vi "DSA Configure AI and AO.vi"(0 "Input  Physical Channel":tag[](array[tag]), 1 "Output Physical Channel":tag[](array[tag]), 2 "Settings Cluster":T1={"Supply Voltage [Vdc]"=0.0, "Max Supply Current [Idc]"=0.0, "Settling Delay"=0.0, "Temp Criteria"=0.0, "Voltage Steps [Vrms]"=[], "User Notes"="", "Config Wave File Path"=path "", "Config Voltage [Vrms]"=0.0, "Channel Configuration List"={"Channel Configuration Cluster"={"Input"=enum."---", "Enable"=FALSE, "User Notes"="", "Voltage Range"=0.0, "Current Range"=2.5}, "Channel Configuration Cluster 2"={"Input"=enum."---", "Enable"=FALSE, "User Notes"="", "Voltage Range"=0.0, "Current Range"=2.5}, "Channel Configuration Cluster 3"={"Input"=enum."---", "Enable"=FALSE, "User Notes"="", "Voltage Range"=0.0, "Current Range"=2.5}, "Channel Configuration Cluster 4"={"Input"=enum."---", "Enable"=FALSE, "User Notes"="", "Voltage Range"=0.0, "Current Range"=2.5}, "Channel Configuration Cluster 5"={"Input"=enum."---", "Enable"=FALSE, "User Notes"="", "Voltage Range"=0.0, "Current Range"=2.5}, "Channel Configuration Cluster 6"={"Input"=enum."---", "Enable"=FALSE, "User Notes"="", "Voltage Range"=0.0, "Current Range"=2.5}, "Channel Configuration Cluster 7"={"Input"=enum."---", "Enable"=FALSE, "User Notes"="", "Voltage Range"=0.0, "Current Range"=2.5}, "Channel Configuration Cluster 8"={"Input"=enum."---", "Enable"=FALSE, "User Notes"="", "Voltage Range"=0.0, "Current Range"=2.5}, "Channel Configuration Cluster 9"={"Input"=enum."---", "Enable"=FALSE, "User Notes"="", "Voltage Range"=0.0, "Current Range"=2.5}, "Channel Configuration Cluster 10"={"Input"=enum."---", "Enable"=FALSE, "User Notes"="", "Voltage Range"=0.0, "Current Range"=2.5}, "Channel Configuration Cluster 11"={"Input"=enum."---", "Enable"=FALSE, "User Notes"="", "Voltage Range"=0.0, "Current Range"=2.5}, "Channel Configuration Cluster 12"={"Input"=enum."---", "Enable"=FALSE, "User Notes"="", "Voltage Range"=0.0, "Current Range"=2.5}, "Channel Configuration Cluster 13"={"Input"=enum."---", "Enable"=FALSE, "User Notes"="", "Voltage Range"=0.0, "Current Range"=2.5}, "Channel Configuration Cluster 14"={"Input"=enum."---", "Enable"=FALSE, "User Notes"="", "Voltage Range"=0.0, "Current Range"=2.5}, "Channel Configuration Cluster 15"={"Input"=enum."---", "Enable"=FALSE, "User Notes"="", "Voltage Range"=0.0, "Current Range"=2.5}, "Channel Configuration Cluster 16"={"Input"=enum."---", "Enable"=FALSE, "User Notes"="", "Voltage Range"=0.0, "Current Range"=2.5}, "Channel Configuration Cluster 17"={"Input"=enum."---", "Enable"=FALSE, "User Notes"="", "Voltage Range"=0.0, "Current Range"=2.5}}, "User Gains"={"Gain 1"=0.0, "Gain 2"=0.0, "Gain 3"=0.0, "Gain 4"=0.0, "Gain 5"=0.0, "Gain 6"=0.0}, "Gains"={"Gain 1"=0.0, "Gain 2"=0.0, "Gain 3"=0.0, "Gain 4"=0.0, "Gain 5"=0.0, "Gain 6"=0.0}, "Gain Array"={"Gain 1"=0.0, "Gain 2"=0.0, "Gain 3"=0.0, "Gain 4"=0.0, "Gain 5"=0.0, "Gain 6"=0.0, "Gain 7"=0.0, "Gain 8"=0.0, "Gain 9"=0.0, "Gain 10"=0.0, "Gain 11"=0.0, "Gain 12"=0.0, "Gain 13"=0.0, "Gain 14"=0.0, "Gain 15"=0.0, "Gain 16"=0.0, "Gain 17"=0.0}, "Wave File Path 1"=path "", "Wave File Path 2"=path "", "Wave File Path 3"=path "", "Wave File Path 4"=path "", "Range"=FALSE, "CF"=FALSE} {"Gain Array"."Gain 17" format="%.2f"; "Gain Array"."Gain 16" format="%.2f"; "Gain Array"."Gain 15" format="%.2f"; "Gain Array"."Gain 14" format="%.2f"; "Gain Array"."Gain 13" format="%.2f"; "Gain Array"."Gain 12" format="%.2f"; "Gain Array"."Gain 11" format="%.2f"; "Gain Array"."Gain 10" format="%.2f"; "Gain Array"."Gain 9" format="%.2f"; "Gain Array"."Gain 8" format="%.2f"; "Gain Array"."Gain 7" format="%.2f"; "Gain Array"."Gain 6" format="%.2f"; "Gain Array"."Gain 5" format="%.2f"; "Gain Array"."Gain 4" format="%.2f"; "Gain Array"."Gain 3" format="%.2f"; "Gain Array"."Gain 2" format="%.2f"; "Gain Array"."Gain 1" format="%.2f"; "Gains"."Gain 6" format="%.2f"; "Gains"."Gain 5" format="%.2f"; "Gains"."Gain 4" format="%.2f"; "Gains"."Gain 3" format="%.2f"; "Gains"."Gain 2" format="%.2f"; "Gains"."Gain 1" format="%.2f"; "User Gains"."Gain 6" format="%.2f"; "User Gains"."Gain 5" format="%.2f"; "User Gains"."Gain 4" format="%.2f"; "User Gains"."Gain 3" format="%.2f"; "User Gains"."Gain 2" format="%.2f"; "User Gains"."Gain 1" format="%.2f"; "Channel Configuration List"."Channel Configuration Cluster 17"."Current Range" items=["1 <500m>"=0.5, "2 <1>"=1.0, "5 <2.5>"=2.5, "10 <5>"=5.0, "20 <10>"=10.0, "50 <25>"=25.0]; "Channel Configuration List"."Channel Configuration Cluster 17"."Voltage Range" items=["1.5 <0.75>"=0.75, "3 <1.5>"=1.5, "6 <3>"=3.0, "10 <5>"=5.0, "15 <7.5>"=7.5, "30 <15>"=15.0, "60 <30>"=30.0, "100 <50>"=50.0, "150 <75>"=75.0, "300 <150>"=150.0, "600 <300>"=300.0, "1000 <500>"=500.0]; "Channel Configuration List"."Channel Configuration Cluster 16"."Current Range" items=["1 <500m>"=0.5, "2 <1>"=1.0, "5 <2.5>"=2.5, "10 <5>"=5.0, "20 <10>"=10.0, "50 <25>"=25.0]; "Channel Configuration List"."Channel Configuration Cluster 16"."Voltage Range" items=["1.5 <0.75>"=0.75, "3 <1.5>"=1.5, "6 <3>"=3.0, "10 <5>"=5.0, "15 <7.5>"=7.5, "30 <15>"=15.0, "60 <30>"=30.0, "100 <50>"=50.0, "150 <75>"=75.0, "300 <150>"=150.0, "600 <300>"=300.0, "1000 <500>"=500.0]; "Channel Configuration List"."Channel Configuration Cluster 15"."Current Range" items=["1 <500m>"=0.5, "2 <1>"=1.0, "5 <2.5>"=2.5, "10 <5>"=5.0, "20 <10>"=10.0, "50 <25>"=25.0]; "Channel Configuration List"."Channel Configuration Cluster 15"."Voltage Range" items=["1.5 <0.75>"=0.75, "3 <1.5>"=1.5, "6 <3>"=3.0, "10 <5>"=5.0, "15 <7.5>"=7.5, "30 <15>"=15.0, "60 <30>"=30.0, "100 <50>"=50.0, "150 <75>"=75.0, "300 <150>"=150.0, "600 <300>"=300.0, "1000 <500>"=500.0]; "Channel Configuration List"."Channel Configuration Cluster 14"."Current Range" items=["1 <500m>"=0.5, "2 <1>"=1.0, "5 <2.5>"=2.5, "10 <5>"=5.0, "20 <10>"=10.0, "50 <25>"=25.0]; "Channel Configuration List"."Channel Configuration Cluster 14"."Voltage Range" items=["1.5 <0.75>"=0.75, "3 <1.5>"=1.5, "6 <3>"=3.0, "10 <5>"=5.0, "15 <7.5>"=7.5, "30 <15>"=15.0, "60 <30>"=30.0, "100 <50>"=50.0, "150 <75>"=75.0, "300 <150>"=150.0, "600 <300>"=300.0, "1000 <500>"=500.0]; "Channel Configuration List"."Channel Configuration Cluster 13"."Current Range" items=["1 <500m>"=0.5, "2 <1>"=1.0, "5 <2.5>"=2.5, "10 <5>"=5.0, "20 <10>"=10.0, "50 <25>"=25.0]; "Channel Configuration List"."Channel Configuration Cluster 13"."Voltage Range" items=["1.5 <0.75>"=0.75, "3 <1.5>"=1.5, "6 <3>"=3.0, "10 <5>"=5.0, "15 <7.5>"=7.5, "30 <15>"=15.0, "60 <30>"=30.0, "100 <50>"=50.0, "150 <75>"=75.0, "300 <150>"=150.0, "600 <300>"=300.0, "1000 <500>"=500.0]; "Channel Configuration List"."Channel Configuration Cluster 12"."Current Range" items=["1 <500m>"=0.5, "2 <1>"=1.0, "5 <2.5>"=2.5, "10 <5>"=5.0, "20 <10>"=10.0, "50 <25>"=25.0]; "Channel Configuration List"."Channel Configuration Cluster 12"."Voltage Range" items=["1.5 <0.75>"=0.75, "3 <1.5>"=1.5, "6 <3>"=3.0, "10 <5>"=5.0, "15 <7.5>"=7.5, "30 <15>"=15.0, "60 <30>"=30.0, "100 <50>"=50.0, "150 <75>"=75.0, "300 <150>"=150.0, "600 <300>"=300.0, "1000 <500>"=500.0]; "Channel Configuration List"."Channel Configuration Cluster 11"."Current Range" items=["1 <500m>"=0.5, "2 <1>"=1.0, "5 <2.5>"=2.5, "10 <5>"=5.0, "20 <10>"=10.0, "50 <25>"=25.0]; "Channel Configuration List"."Channel Configuration Cluster 11"."Voltage Range" items=["1.5 <0.75>"=0.75, "3 <1.5>"=1.5, "6 <3>"=3.0, "10 <5>"=5.0, "15 <7.5>"=7.5, "30 <15>"=15.0, "60 <30>"=30.0, "100 <50>"=50.0, "150 <75>"=75.0, "300 <150>"=150.0, "600 <300>"=300.0, "1000 <500>"=500.0]; "Channel Configuration List"."Channel Configuration Cluster 10"."Current Range" items=["1 <500m>"=0.5, "2 <1>"=1.0, "5 <2.5>"=2.5, "10 <5>"=5.0, "20 <10>"=10.0, "50 <25>"=25.0]; "Channel Configuration List"."Channel Configuration Cluster 10"."Voltage Range" items=["1.5 <0.75>"=0.75, "3 <1.5>"=1.5, "6 <3>"=3.0, "10 <5>"=5.0, "15 <7.5>"=7.5, "30 <15>"=15.0, "60 <30>"=30.0, "100 <50>"=50.0, "150 <75>"=75.0, "300 <150>"=150.0, "600 <300>"=300.0, "1000 <500>"=500.0]; "Channel Configuration List"."Channel Configuration Cluster 9"."Voltage Range" items=["1.5 <0.75>"=0.75, "3 <1.5>"=1.5, "6 <3>"=3.0, "10 <5>"=5.0, "15 <7.5>"=7.5, "30 <15>"=15.0, "60 <30>"=30.0, "100 <50>"=50.0, "150 <75>"=75.0, "300 <150>"=150.0, "600 <300>"=300.0, "1000 <500>"=500.0]; "Channel Configuration List"."Channel Configuration Cluster 9"."Current Range" items=["10m <5m>"=0.005, "20m <10m>"=0.01, "50m <25m>"=0.025, "100m <50m>"=0.05, "200m <100m>"=0.1, "500m <250m>"=0.25, "1 <500m>"=0.5, "2 <1>"=1.0, "5 <2.5>"=2.5]; "Channel Configuration List"."Channel Configuration Cluster 8"."Voltage Range" items=["1.5 <0.75>"=0.75, "3 <1.5>"=1.5, "6 <3>"=3.0, "10 <5>"=5.0, "15 <7.5>"=7.5, "30 <15>"=15.0, "60 <30>"=30.0, "100 <50>"=50.0, "150 <75>"=75.0, "300 <150>"=150.0, "600 <300>"=300.0, "1000 <500>"=500.0]; "Channel Configuration List"."Channel Configuration Cluster 8"."Current Range" items=["10m <5m>"=0.005, "20m <10m>"=0.01, "50m <25m>"=0.025, "100m <50m>"=0.05, "200m <100m>"=0.1, "500m <250m>"=0.25, "1 <500m>"=0.5, "2 <1>"=1.0, "5 <2.5>"=2.5]; "Channel Configuration List"."Channel Configuration Cluster 7"."Voltage Range" items=["1.5 <0.75>"=0.75, "3 <1.5>"=1.5, "6 <3>"=3.0, "10 <5>"=5.0, "15 <7.5>"=7.5, "30 <15>"=15.0, "60 <30>"=30.0, "100 <50>"=50.0, "150 <75>"=75.0, "300 <150>"=150.0, "600 <300>"=300.0, "1000 <500>"=500.0]; "Channel Configuration List"."Channel Configuration Cluster 7"."Current Range" items=["10m <5m>"=0.005, "20m <10m>"=0.01, "50m <25m>"=0.025, "100m <50m>"=0.05, "200m <100m>"=0.1, "500m <250m>"=0.25, "1 <500m>"=0.5, "2 <1>"=1.0, "5 <2.5>"=2.5]; "Channel Configuration List"."Channel Configuration Cluster 6"."Voltage Range" items=["1.5 <0.75>"=0.75, "3 <1.5>"=1.5, "6 <3>"=3.0, "10 <5>"=5.0, "15 <7.5>"=7.5, "30 <15>"=15.0, "60 <30>"=30.0, "100 <50>"=50.0, "150 <75>"=75.0, "300 <150>"=150.0, "600 <300>"=300.0, "1000 <500>"=500.0]; "Channel Configuration List"."Channel Configuration Cluster 6"."Current Range" items=["10m <5m>"=0.005, "20m <10m>"=0.01, "50m <25m>"=0.025, "100m <50m>"=0.05, "200m <100m>"=0.1, "500m <250m>"=0.25, "1 <500m>"=0.5, "2 <1>"=1.0, "5 <2.5>"=2.5]; "Channel Configuration List"."Channel Configuration Cluster 5"."Voltage Range" items=["1.5 <0.75>"=0.75, "3 <1.5>"=1.5, "6 <3>"=3.0, "10 <5>"=5.0, "15 <7.5>"=7.5, "30 <15>"=15.0, "60 <30>"=30.0, "100 <50>"=50.0, "150 <75>"=75.0, "300 <150>"=150.0, "600 <300>"=300.0, "1000 <500>"=500.0]; "Channel Configuration List"."Channel Configuration Cluster 5"."Current Range" items=["10m <5m>"=0.005, "20m <10m>"=0.01, "50m <25m>"=0.025, "100m <50m>"=0.05, "200m <100m>"=0.1, "500m <250m>"=0.25, "1 <500m>"=0.5, "2 <1>"=1.0, "5 <2.5>"=2.5]; "Channel Configuration List"."Channel Configuration Cluster 4"."Voltage Range" items=["1.5 <0.75>"=0.75, "3 <1.5>"=1.5, "6 <3>"=3.0, "10 <5>"=5.0, "15 <7.5>"=7.5, "30 <15>"=15.0, "60 <30>"=30.0, "100 <50>"=50.0, "150 <75>"=75.0, "300 <150>"=150.0, "600 <300>"=300.0, "1000 <500>"=500.0]; "Channel Configuration List"."Channel Configuration Cluster 4"."Current Range" items=["10m <5m>"=0.005, "20m <10m>"=0.01, "50m <25m>"=0.025, "100m <50m>"=0.05, "200m <100m>"=0.1, "500m <250m>"=0.25, "1 <500m>"=0.5, "2 <1>"=1.0, "5 <2.5>"=2.5]; "Channel Configuration List"."Channel Configuration Cluster 3"."Voltage Range" items=["1.5 <0.75>"=0.75, "3 <1.5>"=1.5, "6 <3>"=3.0, "10 <5>"=5.0, "15 <7.5>"=7.5, "30 <15>"=15.0, "60 <30>"=30.0, "100 <50>"=50.0, "150 <75>"=75.0, "300 <150>"=150.0, "600 <300>"=300.0, "1000 <500>"=500.0]; "Channel Configuration List"."Channel Configuration Cluster 3"."Current Range" items=["10m <5m>"=0.005, "20m <10m>"=0.01, "50m <25m>"=0.025, "100m <50m>"=0.05, "200m <100m>"=0.1, "500m <250m>"=0.25, "1 <500m>"=0.5, "2 <1>"=1.0, "5 <2.5>"=2.5]; "Channel Configuration List"."Channel Configuration Cluster 2"."Voltage Range" items=["1.5 <0.75>"=0.75, "3 <1.5>"=1.5, "6 <3>"=3.0, "10 <5>"=5.0, "15 <7.5>"=7.5, "30 <15>"=15.0, "60 <30>"=30.0, "100 <50>"=50.0, "150 <75>"=75.0, "300 <150>"=150.0, "600 <300>"=300.0, "1000 <500>"=500.0]; "Channel Configuration List"."Channel Configuration Cluster 2"."Current Range" items=["10m <5m>"=0.005, "20m <10m>"=0.01, "50m <25m>"=0.025, "100m <50m>"=0.05, "200m <100m>"=0.1, "500m <250m>"=0.25, "1 <500m>"=0.5, "2 <1>"=1.0, "5 <2.5>"=2.5]; "Channel Configuration List"."Channel Configuration Cluster"."Voltage Range" items=["1.5 <0.75>"=0.75, "3 <1.5>"=1.5, "6 <3>"=3.0, "10 <5>"=5.0, "15 <7.5>"=7.5, "30 <15>"=15.0, "60 <30>"=30.0, "100 <50>"=50.0, "150 <75>"=75.0, "300 <150>"=150.0, "600 <300>"=300.0, "1000 <500>"=500.0]; "Channel Configuration List"."Channel Configuration Cluster"."Current Range" items=["10m <5m>"=0.005, "20m <10m>"=0.01, "50m <25m>"=0.025, "100m <50m>"=0.05, "200m <100m>"=0.1, "500m <250m>"=0.25, "1 <500m>"=0.5, "2 <1>"=1.0, "5 <2.5>"=2.5]; "Settling Delay" min=0.0 format="%<%H:%M:%S>t"}, 3 "Wave Generator Cluster":T7 {"Signal Type" items=["Calibration Sine", "Sine", "Linear Chirp", "Log Chirp", "Pink Noise", "Periodic Random Noise", "Uniform White Noise", "Gaussian White Noise", "11db4816 Wave File"]}, 4 "Sampling Rate [Hz]":dbl=48000.0, 5 "Error In":errorcluster, 6 "Voltage Step":dbl, 7 "Run Mode (Manual = True)":bool, 8 "Block Lenght (50ms)":dbl) -> (11 "actual sample rate":dbl, 12 "Waveform":waveform(dbl)[][](array[waveform]), 13 "samples per channel":i32=-1, 14 "AI Task ID Out":refnum<k21>, 15 "AO Task ID Out":refnum<k21>[](array[refnum]), 17 "Waveform Duration":dbl, 18 "Step Delay":dbl, 19 "Error out":errorcluster)   [LabVIEW 2021]
uses:
  Controls/Wave Generator Control.ctl
  Controls/Settings Control.ctl
  Controls/Channel Configuration List.ctl
  Controls/Channel Configuration Cluster.ctl
  Controls/Channel Configuration Cluster High Current.ctl
  Controls/Gain Averages.ctl
  Controls/Gain Array.ctl
  <vilib>/DAQmx/read.llb/DAQmx Read (Analog 1D DBL NChan 1Samp).vi
  <vilib>/DAQmx/write.llb/DAQmx Write (Analog 1D Wfm NChan NSamp).vi
  <vilib>/DAQmx/read.llb/DAQmx Read (Analog 1D Wfm NChan NSamp).vi
  <vilib>/DAQmx/create/channels.llb/DAQmx Create Channel (AO-Voltage-Basic).vi
  <vilib>/DAQmx/configure/timing.llb/DAQmx Timing (Sample Clock).vi
  <vilib>/DAQmx/create/channels.llb/DAQmx Create Channel (AI-Voltage-Basic).vi
  <vilib>/DAQmx/create/channels.llb/DAQmx Create Channel (AI-Temperature-Thermocouple).vi
  <vilib>/DAQmx/miscellaneous.llb/DAQmx Fill In Error Info.vi
  <vilib>/DAQmx/configure/trigger.llb/DAQmx Start Trigger (Digital Edge).vi
  <resource>/objmgr/daqmx.rc
panel:
  out "Temperature Data":dbl[](array[numeric])
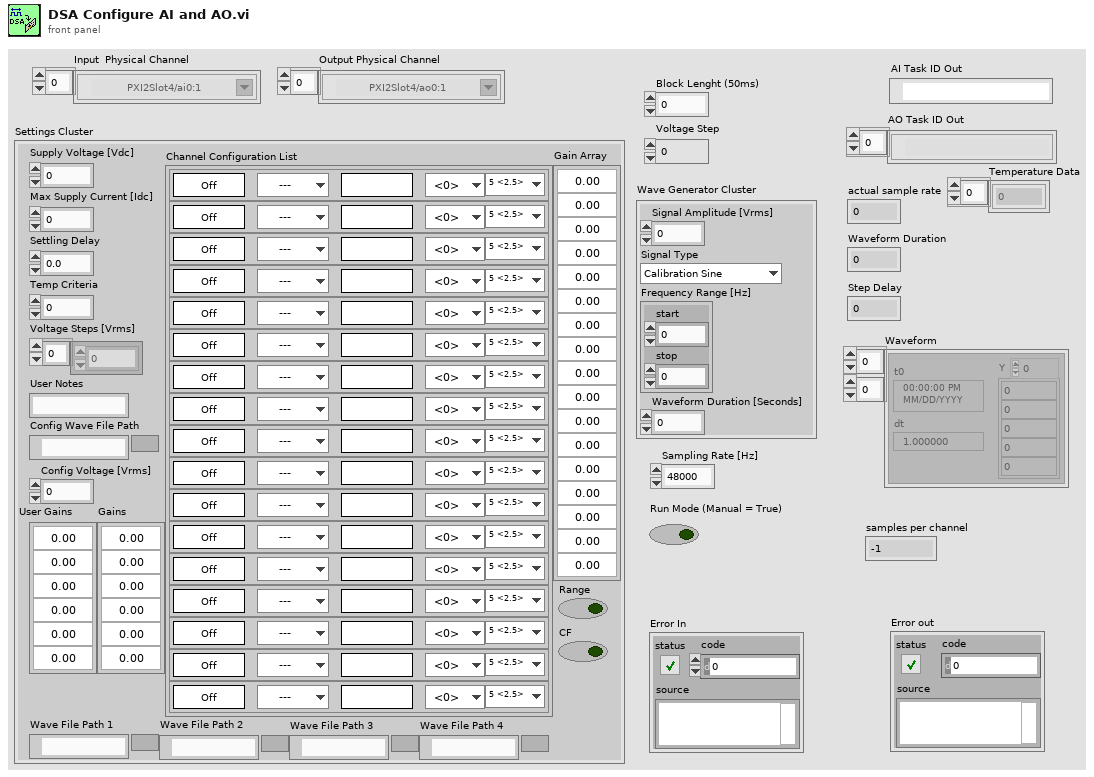
[diagram p1: front panel]
types:
  T1 = typedef "Settings Control.ctl" = cluster{"Supply Voltage [Vdc]":sgl, "Max Supply Current [Idc]":sgl, "Settling Delay":dbl, "Temp Criteria":sgl, "Voltage Steps [Vrms]":sgl[], "User Notes":string, "Config Wave File Path":path, "Config Voltage [Vrms]":sgl, "Channel Configuration List":T2, "User Gains":T5, "Gains":T5, "Gain Array":T6, "Wave File Path 1":path, "Wave File Path 2":path, "Wave File Path 3":path, "Wave File Path 4":path, "Range":bool, "CF":bool}
  T2 = typedef "Channel Configuration List.ctl" = cluster{"Channel Configuration Cluster":T3, "Channel Configuration Cluster 2":T3, "Channel Configuration Cluster 3":T3, "Channel Configuration Cluster 4":T3, "Channel Configuration Cluster 5":T3, "Channel Configuration Cluster 6":T3, "Channel Configuration Cluster 7":T3, "Channel Configuration Cluster 8":T3, "Channel Configuration Cluster 9":T3, "Channel Configuration Cluster 10":T4, "Channel Configuration Cluster 11":T4, "Channel Configuration Cluster 12":T4, "Channel Configuration Cluster 13":T4, "Channel Configuration Cluster 14":T4, "Channel Configuration Cluster 15":T4, "Channel Configuration Cluster 16":T4, "Channel Configuration Cluster 17":T4}
  T3 = typedef "Channel Configuration Cluster.ctl" = cluster{"Input":enum16{"---", "1", "1 AVG", "2", "2 AVG", "3", "3 AVG", "4", "4 AVG"}, "Enable":bool, "User Notes":string, "Voltage Range":dbl, "Current Range":dbl}
  T4 = typedef "Channel Configuration Cluster High Current.ctl" = cluster{"Input":enum16{"---", "1", "1 AVG", "2", "2 AVG", "3", "3 AVG", "4", "4 AVG"}, "Enable":bool, "User Notes":string, "Voltage Range":dbl, "Current Range":dbl}
  T5 = typedef "Gain Averages.ctl" = cluster{"Gain 1":dbl, "Gain 2":dbl, "Gain 3":dbl, "Gain 4":dbl, "Gain 5":dbl, "Gain 6":dbl}
  T6 = typedef "Gain Array.ctl" = cluster{"Gain 1":dbl, "Gain 2":dbl, "Gain 3":dbl, "Gain 4":dbl, "Gain 5":dbl, "Gain 6":dbl, "Gain 7":dbl, "Gain 8":dbl, "Gain 9":dbl, "Gain 10":dbl, "Gain 11":dbl, "Gain 12":dbl, "Gain 13":dbl, "Gain 14":dbl, "Gain 15":dbl, "Gain 16":dbl, "Gain 17":dbl}
  T7 = typedef "Wave Generator Control.ctl" = cluster{"Signal Amplitude [Vrms]":dbl, "Signal Type":u16, "Frequency Range [Hz]":cluster{"start":dbl, "stop":dbl}, "Waveform Duration [Seconds]":dbl}
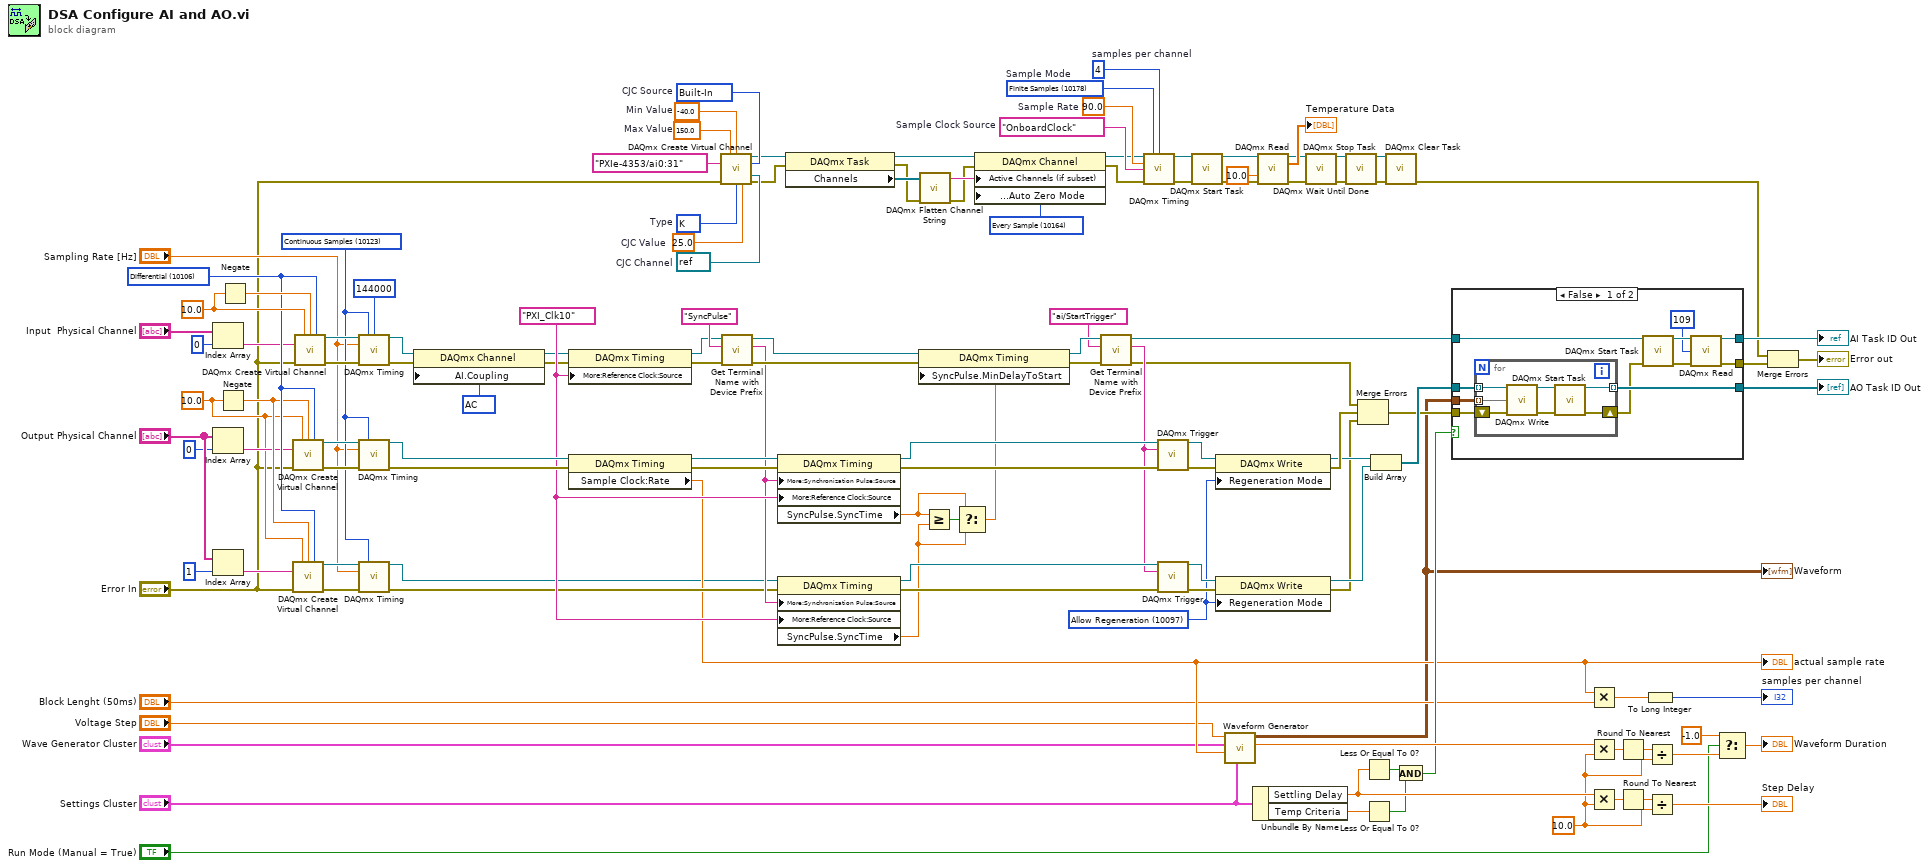
[diagram p0: block diagram]
diagram:
  w15 = 10045 items=["AC"=10045, "DC"=10050, "GND"=10066] ("AI.Coupling")
  w18 = 4  # samples per channel
  w24 = 10164 items=["None"=10230, "Once"=10244, "Every Sample"=10164] ("Auto Zero Mode")
  w42 = refnum<k21> refnum  # CJC Channel
  w37 = 10200 items=["Built-In"=10200, "Constant Value"=10116, "Channel"=10113]  # CJC Source
  w38 = -40.0  # Min Value
  w39 = 150.0  # Max Value
  w41 = 25.0  # CJC Value
  w40 = 10073 items=["J"=10072, "K"=10073, "N"=10077, "R"=10082, "S"=10085, "T"=10086, "B"=10047, "E"=10055]  # Type
  w34 = 90.0  # Sample Rate
  w35 = tag "OnboardClock"  # Sample Clock Source
  w36 = 10178 items=["Finite Samples"=10178, "Continuous Samples"=10123, "Hardware Timed Single Point"=12522]  # Sample Mode
  w76 = 10.0 ("y")
  w90 = 10097 items=["Allow Regeneration"=10097, "Do Not Allow Regeneration"=10158] ("RegenMode")
  w50 = 10.0 ("maximum value")
  w97 = 10106 items=["default"=-1, "RSE"=10083, "NRSE"=10078, "Differential"=10106, "Pseudodifferential"=12529] ("input terminal configuration")
  w100 = 10.0 ("maximum value")
  w104 = tag "PXI_Clk10" ("RefClk.Src")
  w113 = 10123 items=["Finite Samples"=10178, "Continuous Samples"=10123, "Hardware Timed Single Point"=12522] ("Sample Mode")
  n1 = Index Array(array="Input  Physical Channel", index=0) -> (element=w57:tag)
  n2 = Index Array(array="Output Physical Channel", index=0) -> (element=w63:tag)
  n3 = Index Array(array="Output Physical Channel", index=1) -> (element=w62:tag)
  n4 = Negate(x=w50) -> (-x=w96:dbl)
  n5 = Negate(x=w100) -> (-x=w99:dbl)
  n6 = call-poly <vilib>:"DAQmx Create Virtual Channel.vi"("maximum value"=w50, "minimum value"=w96, "output terminal configuration"=w97, "physical channels"=w63, "error in"="Error In") -> ("task out"=w125:refnum<k21>, "error out"=w126:errorcluster)  [unwired: 9 in]
  n7 = call-poly <vilib>:"DAQmx Create Virtual Channel.vi"("maximum value"=w50, "minimum value"=w96, "output terminal configuration"=w97, "physical channels"=w62, "error in"="Error In") -> ("task out"=w115:refnum<k21>, "error out"=w114:errorcluster)  [unwired: 9 in]
  n8 = call-poly <vilib>:"DAQmx Create Virtual Channel.vi"("maximum value"=w100, "minimum value"=w99, "input terminal configuration"=w97, "physical channels"=w57, "error in"="Error In") -> ("task out"=w128:refnum<k21>, "error out"=w127:errorcluster)  [unwired: 9 in]
  n9 = call-poly <vilib>:"DAQmx Timing.vi"("task/channels in"=w128, "sample mode"=w113, "samples per channel"=144000, "rate"="Sampling Rate [Hz]", "error in"=w127) -> ("task out"=w12:refnum<k21>, "error out"=w14:errorcluster)  [unwired: 9 in]
  n10 = call-poly <vilib>:"DAQmx Timing.vi"("task/channels in"=w125, "sample mode"=w113, "rate"="Sampling Rate [Hz]", "error in"=w126) -> ("task out"=w119:refnum<k21>, "error out"=w117:errorcluster)  [unwired: 10 in]
  n11 = call-poly <vilib>:"DAQmx Timing.vi"("task/channels in"=w115, "sample mode"=w113, "rate"="Sampling Rate [Hz]", "error in"=w114) -> ("task out"=w16:refnum<k21>, "error out"=w102:errorcluster)  [unwired: 10 in]
  n12 = property class="DAQmx Channel"(reference=w12, error in=w14, "AI.Coupling"=w15) -> (reference out=w11:refnum<k21>, error out=w13:errorcluster)
  n13 = property class="DAQmx Timing"(reference=w11, error in=w13, "More:Reference Clock:Source"=w104) -> (reference out=w108:refnum<k21>, error out=w107:errorcluster)
  n14 = property class="DAQmx Timing"(reference=w119, error in=w117) -> (reference out=w118:refnum<k21>, error out=w116:errorcluster, "Sample Clock:Rate"=w68:dbl)
  "actual sample rate" <- w68
  n15 = call-poly <vilib>:"DAQmx Create Virtual Channel.vi"("maximum value"=w39, "minimum value"=w38, "physical channels"=tag "PXIe-4353/ai0:31" ("Physical Channel"), "cjc source"=w37, "cjc channel"=w42, "error in"="Error In", "thermocouple type"=w40, "cjc value"=w41) -> ("task out"=w33:refnum<k21>, "error out"=w31:errorcluster)  [unwired: 6 in]
  n16 = call "Get Terminal Name with Device Prefix.vi"("error in"=w107, "Local Terminal Name"="SyncPulse", "task/channels in"=w108) -> ("error out"=w105:errorcluster, "Terminal Name with Device Prefix"=w103:tag, "task out"=w106:refnum<k21>)  [unwired: 6 in]
  n17 = property class="DAQmx Timing"(reference=w118, error in=w116, "More:Synchronization Pulse:Source"=w103, "More:Reference Clock:Source"=w104) -> (reference out=w124:refnum<k21>, error out=w123:errorcluster, "SyncPulse.SyncTime"=w88:dbl)
  n18 = property class="DAQmx Timing"(reference=w16, error in=w102, "More:Synchronization Pulse:Source"=w103, "More:Reference Clock:Source"=w104) -> (reference out=w112:refnum<k21>, error out=w111:errorcluster, "SyncPulse.SyncTime"=w86:dbl)
  n19 = property class="DAQmx Task"(reference=w33, error in=w31) -> (reference out=w29:refnum<k21>, error out=w26:errorcluster, "Channels"=w28:refnum<k21>[])
  n20 = call <vilib>:"DAQmx Flatten Channel String.vi"("names in"=w28, "error in"=w26) -> ("names out"=w27:string, "error out"=w25:errorcluster)  [unwired: 12 in]
  n21 = Greater Or Equal?(x=w88, y=w86) -> (x >= y?=w87:bool)
  n22 = Select(t=w88, s=w87, f=w86) -> (s? t:f=w85:dbl)
  n23 = property class="DAQmx Timing"(reference=w106, error in=w105, "SyncPulse.MinDelayToStart"=w85) -> (reference out=w122:refnum<k21>, error out=w121:errorcluster)
  n24 = property class="DAQmx Channel"(reference=w29, error in=w25, "Active Channels (if subset)"=w27, "Analog Input:General Properties:Advanced:High Accuracy Settings:Auto Zero Mode"=w24) -> (reference out=w32:refnum<k21>, error out=w30:errorcluster)
  n25 = call "Get Terminal Name with Device Prefix.vi"("error in"=w121, "Local Terminal Name"="ai/StartTrigger", "task/channels in"=w122) -> ("error out"=w101:errorcluster, "Terminal Name with Device Prefix"=w110:tag, "task out"=w55:refnum<k21>)  [unwired: 6 in]
  n26 = call-poly <vilib>:"DAQmx Timing.vi"("task/channels in"=w32, "sample mode"=w36, "samples per channel"=w18, "rate"=w34, "source"=w35, "error in"=w30) -> ("task out"=w43:refnum<k21>, "error out"=w23:errorcluster)  [unwired: 8 in]
  n27 = call-poly <vilib>:"DAQmx Trigger.vi"("task/channels in"=w124, "source"=w110, "error in"=w123) -> ("task out"=w95:refnum<k21>, "error out"=w94:errorcluster)  [unwired: 11 in]
  n28 = call-poly <vilib>:"DAQmx Trigger.vi"("task/channels in"=w112, "source"=w110, "error in"=w111) -> ("task out"=w92:refnum<k21>, "error out"=w91:errorcluster)  [unwired: 11 in]
  n29 = call <vilib>:"DAQmx Start Task.vi"("task/channels in"=w43, "error in"=w23) -> ("task out"=w21:refnum<k21>, "error out"=w20:errorcluster)  [unwired: 12 in]
  n30 = property class="DAQmx Write"(reference=w95, error in=w94, "Regeneration Mode"=w90) -> (reference out=w74:refnum<k21>, error out=w93:errorcluster)
  n31 = property class="DAQmx Write"(reference=w92, error in=w91, "Regeneration Mode"=w90) -> (reference out=w73:refnum<k21>, error out=w71:errorcluster)
  n32 = call "Waveform Generator.vi"("Settings Cluster"="Settings Cluster", "Actual Sample Rate"=w68, "Wave Generator Cluster"="Wave Generator Cluster", "Signal Amplitude [Vrms]"="Voltage Step") -> ("Actual Waveform Duration [Seconds]"=w75:dbl, "Waveform Out"=w51:waveform(dbl)[][])  [unwired: 5 in, 1 out]
  "Waveform" <- w51
  n33 = Unbundle By Name("Settings Cluster") -> ("Settling Delay"=w81:dbl, "Temp Criteria"=w80:sgl)
  n34 = call-poly <vilib>:"DAQmx Read.vi"("task/channels in"=w21, "timeout"=10.0, "error in"=w20) -> ("task out"=w7:refnum<k21>, "data"=→"Temperature Data":dbl[], "error out"=w5:errorcluster)  [unwired: 10 in]
  n35 = call <vilib>:"DAQmx Wait Until Done.vi"("task/channels in"=w7, "error in"=w5) -> ("task out"=w6:refnum<k21>, "error out"=w4:errorcluster)  [unwired: 12 in]
  n36 = call <vilib>:"DAQmx Stop Task.vi"("task/channels in"=w6, "error in"=w4) -> ("task out"=w45:refnum<k21>, "error out"=w44:errorcluster)  [unwired: 12 in]
  n37 = Merge Errors(w101, w93, w71) -> (w56:errorcluster)
  n38 = Less Or Equal To 0?(x=w81) -> (x <= 0?=w84:bool)
  n39 = Less Or Equal To 0?(x=w80) -> (x <= 0?=w79:bool)
  n40 = Build Array(w74, w73) -> (w72:refnum<k21>[])
  n41 = call <vilib>:"DAQmx Clear Task.vi"("task in"=w45, "error in"=w44) -> ("error out"=w8:errorcluster)  [unwired: 13 in]
  n42 = And(x=w84, y=w79) -> (x .and. y?=w70:bool)
  n43 = case shown="False" w70 {
    tunnel: w72 -> [w139 w149]
    tunnel: w56 -> [w138 w147]
    tunnel: w55 -> [w132 w148]
    tunnel: w51 -> [w137 _]
    tunnel: [w136 w149] -> w66
    tunnel: [w130 w148] -> w54
    tunnel: [w129 w147] -> w53
    frame False {
      n44 = for {
        tunnel: w139 -> [w146] mode=indexing
        tunnel: w137 -> [w144] mode=indexing
        tunnel: [w141] -> w136 mode=indexing
        shift-right: [w140] -> w131
        shift-left: w138 -> [w145]
        n45 = call-poly <vilib>:"DAQmx Write.vi"("task/channels in"=w146, "data"=w144, "error in"=w145) -> ("task out"=w143:refnum<k21>, "error out"=w142:errorcluster)  [unwired: 10 in, 1 out]
        n46 = call <vilib>:"DAQmx Start Task.vi"("task/channels in"=w143, "error in"=w142) -> ("task out"=w141:refnum<k21>, "error out"=w140:errorcluster)  [unwired: 12 in]
      }
      n47 = call <vilib>:"DAQmx Start Task.vi"("task/channels in"=w132, "error in"=w131) -> ("task out"=w134:refnum<k21>, "error out"=w135:errorcluster)  [unwired: 12 in]
      n48 = call-poly <vilib>:"DAQmx Read.vi"("task/channels in"=w134, "number of samples per channel"=109, "error in"=w135) -> ("task out"=w130:refnum<k21>, "error out"=w129:errorcluster)  [unwired: 10 in, 1 out]
    }
    frame True {
    }
  }
  "AO Task ID Out" <- w66
  "AI Task ID Out" <- w54
  n49 = Multiply(x=w68, y="Block Lenght (50ms)") -> (x*y=w89:dbl)
  n50 = Multiply(x=w75, y=w76) -> (x*y=w77:dbl)
  n51 = Multiply(x=w81, y=w76) -> (x*y=w83:dbl)
  n52 = Round To Nearest(number=w77) -> (nearest integer value=w78:dbl)
  n53 = Round To Nearest(number=w83) -> (nearest integer value=w82:dbl)
  n54 = To Long Integer(number=w89) -> (32bit integer=→"samples per channel":i32)
  n55 = Divide(x=w78, y=w76) -> (x/y=w48:dbl)
  n56 = Divide(x=w82, y=w76) -> (x/y=→"Step Delay":dbl)
  n57 = Select(t=-1.0, s="Run Mode (Manual = True)", f=w48) -> (s? t:f=→"Waveform Duration":dbl)
  n58 = Merge Errors(w8, w53) -> (→"Error out":errorcluster)
